vi "Plugin Loader Launcher.vi"(10 "Loader Name Override":string, 11 "Plugin Loader Path Override":path) -> (0 "error out":errorcluster)   [LabVIEW 2021, in "CIF Engine Launch.lvlib"]
uses:
  CIF Engine Launch.lvlib
  <vilib>/Utility/LVLibp/NI_PackedLibraryUtility.lvlib
  363d3bde-6874-4068-849e-62e045d4c070.vi
  CIFUtilities/CIFConfigurationFile/CIF Configuration File.lvlib
  CIFUtilities/CIFConfigurationFile/typedef/Location Type.ctl
  CIFUtilities/CIFLogs/CIFLogs.lvlib
  CIFUtilities/CIFLogs/Typedef/Message Type.ctl
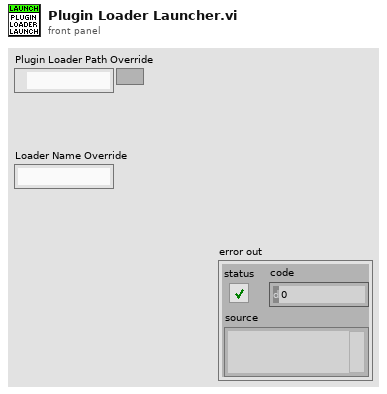
[diagram p1: front panel]
types:
  T1 = typedef "CIF Configuration File.lvlib/Location Type.ctl" = enum16{"Config File", "Manager", "Protos", "Plugins", "UI Plugins", "Logs", "Orchestrations", "Loaders"}
  T2 = typedef "CIFLogs.lvlib/Message Type.ctl" = enum16{"Error", "Information", "Print Terminal", "Configuration"}
  T3 = enum32{"Invalid", "Standard", "Closed", "Hidden", "Minimized", "Maximized"}
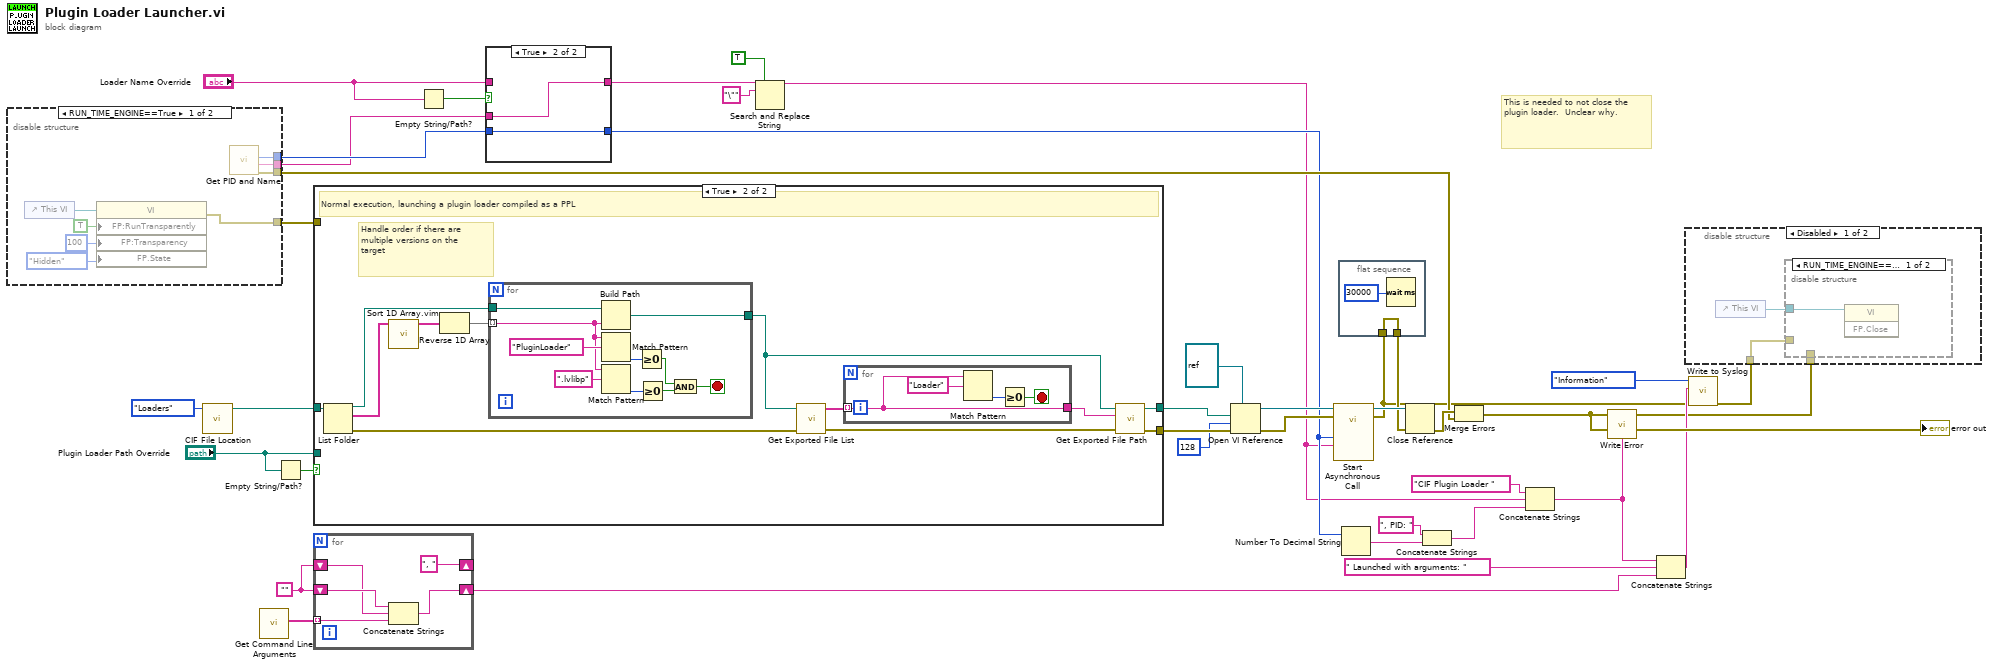
[diagram p0: block diagram]
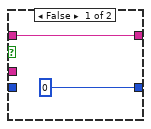
[diagram p4: hidden frame]
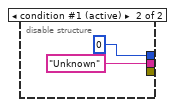
[diagram p6: hidden frame]
diagram:
  w11 = ""
  # "This is needed to not close the plugin loader.  Unclear why."
  n1 = disable-structure shown="RUN_TIME_ENGINE==True" {
    disable-tunnel: [w46 _] -> w24
    disable-tunnel: [w42 u32 0 ("pid")] -> w22
    disable-tunnel: [w41 "Unknown" ("launcher_name")] -> w21
    disable-tunnel: [w40 _] -> w27
    frame condition #0 {
      n2 = control-ref of="This VI"() -> (w47:refnum<vi>)
      n3 = property class="VI"(reference=w47, "FP:RunTransparently"=TRUE ("Front Panel Window:Run VI Transparently"), "FP:Transparency"=u8 100 ("Front Panel Window:Transparency"), "FP.State"=T3."Hidden" ("Front Panel Window:State")) -> (error out=w46:errorcluster)  [unwired: 1 in, 1 out]
      n4 = call "Get PID and Name.vi"() -> ("error out"=w40:errorcluster, "Name"=w41:string, "PID"=w42:u32)  [unwired: 9 in]
    }
    frame condition #1 (active) {
    }
  }
  n5 = call "CIF File Location.vi"("LocationType"=Location_Type."Loaders") -> ("Location"=w33:path)  [unwired: 10 in]
  n6 = call <vilib>:"Get Command Line Arguments.vi"() -> ("arguments"=w8:string[])  [unwired: 9 in, 2 out]
  n7 = Empty String/Path?(string/path="Plugin Loader Path Override") -> (empty?=w26:bool)
  n8 = case shown="True" w26 {
    tunnel: [w50 w55] -> w39
    tunnel: [_ w54] -> w38
    tunnel: w33 -> [_ w52]
    tunnel: "Plugin Loader Path Override" -> [w50 _]
    tunnel: w24 -> [_ _]
    frame False {
      # "Test where Plugin Loader is VI or qualified path to PPL is manually provided"
    }
    frame True {
      # "Handle order if there are multiple versions on the target"
      # "Normal execution, launching a plugin loader compiled as a PPL"
      n9 = List Folder(path=w52) -> (path out=w61:path, filenames=w59:string[], error out=w62:errorcluster)  [unwired: 3 in, 1 out]
      n10 = call "Sort 1D Array.vim"("unsorted array"=w59) -> ("sorted array"=w58:string[])  [unwired: 10 in]
      n11 = Reverse 1D Array(array=w58) -> (reversed array=w57:string[])
      n12 = for {
        tunnel: w57 -> [w72] mode=indexing
        tunnel: [w73] -> w60
        tunnel: w61 -> [w74]
        stop <- w67 stop-if-true
        n13 = Build Path(base path=w74, name or relative path=w72) -> (appended path=w73:path)
        n14 = Match Pattern(string=w72, regular expression="PluginLoader") -> (offset past match=w76:i32)  [unwired: 1 in, 3 out]
        n15 = Match Pattern(string=w72, regular expression=".lvlibp") -> (offset past match=w70:i32)  [unwired: 1 in, 3 out]
        n16 = Greater Or Equal To 0?(x=w76) -> (x >= 0?=w68:bool)
        n17 = Greater Or Equal To 0?(x=w70) -> (x >= 0?=w69:bool)
        n18 = And(x=w68, y=w69) -> (x .and. y?=w67:bool)
      }
      n19 = call <vilib>:"Get Exported File List.vi"("error in (no error)"=w62, "packed library path"=w60) -> ("error out"=w51:errorcluster, "qualified names"=w56:string[])  [unwired: 7 in, 1 out]
      n20 = for {
        tunnel: w56 -> [w63] mode=indexing
        tunnel: [w63] -> w53
        stop <- w65 stop-if-true
        n21 = Match Pattern(string=w63, regular expression="Loader") -> (offset past match=w66:i32)  [unwired: 1 in, 3 out]
        n22 = Greater Or Equal To 0?(x=w66) -> (x >= 0?=w65:bool)
      }
      n23 = call <vilib>:"Get Exported File Path.vi"("error in (no error)"=w51, "qualified name"=w53, "packed library path"=w60) -> ("error out"=w54:errorcluster, "path"=w55:path)  [unwired: 7 in]
    }
  }
  n24 = for {
    tunnel: w8 -> [w81] mode=indexing
    shift-right: [w80] -> w12
    shift-left: w11 -> [w78]
    shift-right: [", "] -> _
    shift-left: w11 -> [w77]
    n25 = Concatenate Strings(w78, w77, w81) -> (w80:string)
  }
  n26 = Empty String/Path?(string/path="Loader Name Override") -> (empty?=w23:bool)
  n27 = case shown="True" w23 {
    tunnel: w22 -> [_ w85]
    tunnel: w21 -> [_ w84]
    tunnel: "Loader Name Override" -> [w83 _]
    tunnel: [u32 0 ("pid") w85] -> w17
    tunnel: [w83 w84] -> w7
    frame False {
    }
    frame True {
    }
  }
  n28 = Search and Replace String(replace all?=TRUE ("replace all? (F)"), input string=w7, search string="\"") -> (result string=w4:string)  [unwired: 5 in, 3 out]
  n29 = Open VI Reference(type specifier VI Refnum (for type only)=refnum<vi> refnum, vi path=w39, options=128, error in (no error)=w38) -> (vi reference=w36:refnum<vi>, error out=w35:errorcluster)  [unwired: 2 in]
  n30 = call-by-ref "Start Asynchronous Call"(reference=w36, error in=w35, "launcher_name"=w4, "pid"=w17) -> (reference out=w34:refnum<vi>, error out=w2:errorcluster)  [unwired: 10 in]
  n31 = flat-sequence {
    tunnel: w2 -> [w86]
    tunnel: [w86] -> w3
    frame #0 {
      n32 = Wait (ms)(milliseconds to wait=u32 30000) -> ()  [unwired: 1 out]
    }
  }
  n33 = Number To Decimal String(number=w17) -> (decimal integer string=w16:string)  [unwired: 1 in]
  n34 = Close Reference(reference=w34, error in (no error)=w3) -> (error out=w29:errorcluster)
  n35 = Concatenate Strings(", PID: " ("string"), w16) -> (w15:string)
  n36 = Merge Errors(w29, w27) -> (w28:errorcluster)
  "error out" <- w28
  n37 = Concatenate Strings("CIF Plugin Loader " ("Plugin Name"), w4, w15) -> (w14:string)
  n38 = call "Write Error.vi"("error in (no error)"=w28, "Plugin Name"=w14) -> ("cleared error"=w1:errorcluster)  [unwired: 2 in]
  n39 = Concatenate Strings(w14, " Launched with arguments: " ("message"), w12) -> (w18:string)
  n40 = call "Write to Syslog.vi"("error in (no error)"=w2, "message"=w18, "CIF Message Type"=Message_Type."Information") -> ("error out"=w32:errorcluster)  [unwired: 8 in]
  n41 = disable-structure shown="Disabled" {
    disable-tunnel: w32 -> [w89 _]
    disable-tunnel: w1 -> [w88 _]
    frame Disabled {
      n42 = control-ref of="This VI"() -> (w90:refnum<vi>)
      n43 = disable-structure shown="RUN_TIME_ENGINE==True" {
        disable-tunnel: w90 -> [w91 _]
        disable-tunnel: w89 -> [_ _]
        disable-tunnel: w88 -> [_ _]
        frame condition #0 {
          n44 = invoke class="VI" method="FP.Close"(reference=w91) -> ()  [unwired: 2 in, 3 out]
        }
        frame condition #1 (active) {
        }
      }
    }
    frame Enabled {
    }
  }
